vi "Fit.vi"(8 "error in (no error)":errorcluster caption="entrée d'erreur (pas d'erreur)", 9 "y":string[][](array[string]), 10 "X":string[][](array[string]), 11 "FunctionTransformer.lvclass":refnum<class "FunctionTransformer.lvclass">) -> (0 "error in (no error)":errorcluster caption="entrée d'erreur (pas d'erreur)", 2 "String Data":string, 3 "FunctionTransformer.lvclass":refnum<class "FunctionTransformer.lvclass">)   [LabVIEW 2020, in "FunctionTransformer.lvclass"]
doc: "Fit transformer by checking X.\n\nIf validate is True, X will be checked.\n\nReturns : \n\n- String : OK"
uses:
  FunctionTransformer.lvclass
  FunctionTransformer.lvclass/FunctionTransformer.ctl
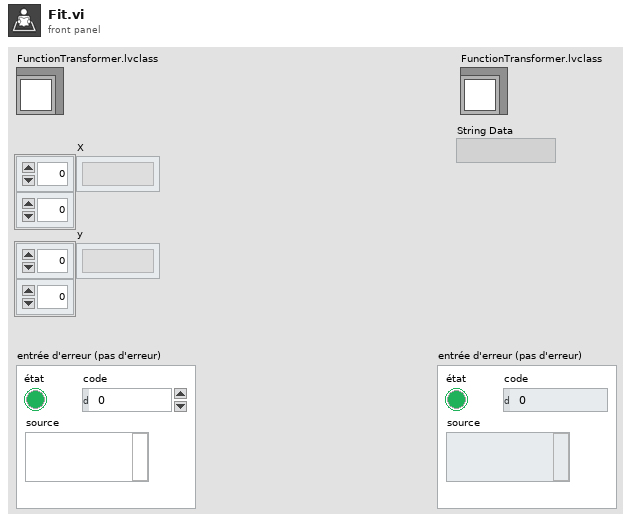
[diagram p1: front panel]
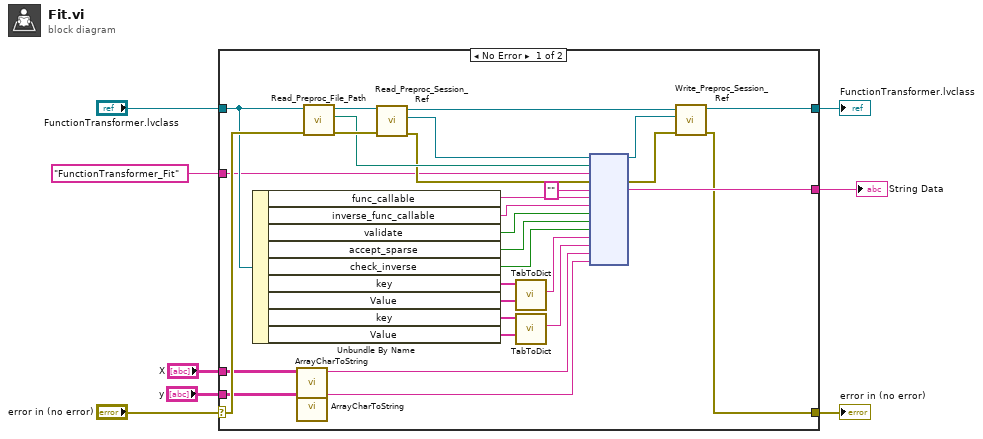
[diagram p0: block diagram]
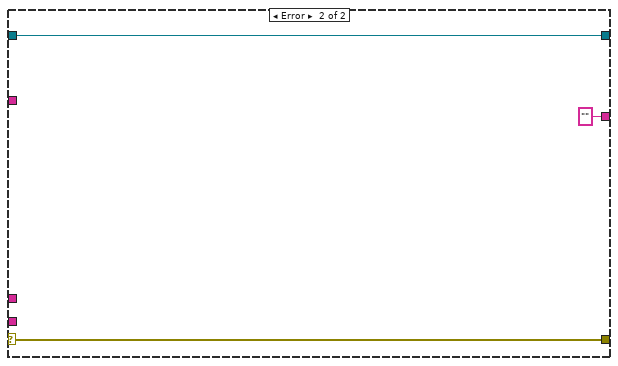
[diagram p2: hidden frame]
diagram:
  n1 = case shown="No Error" "error in (no error)" {
    selector: "error in (no error)" -> [w29 w41]
    tunnel: [w19 w41] -> w7
    tunnel: [w21 w40] -> w5
    tunnel: "FunctionTransformer.lvclass" -> [w28 w40]
    tunnel: "FunctionTransformer_Fit" ("Fonction") -> [w22 _]
    tunnel: [w20 ""] -> w3
    tunnel: "X" -> [w12 _]
    tunnel: "y" -> [w11 _]
    frame No Error {
      n2 = Unbundle By Name(w28) -> ("func_callable"=w27:string, "inverse_func_callable"=w26:string, "validate"=w25:bool, "accept_sparse"=w24:bool, "check_inverse"=w23:bool, "key"=w18:string[], "Value"=w17:string[], "key"=w16:string[], "Value"=w15:string[])
      n3 = call "ArrayCharToString.vi"("TAB"=w12) -> ("Instruction"=w10:string)  [unwired: 10 in]
      n4 = call "ArrayCharToString.vi"("TAB"=w11) -> ("Instruction"=w9:string)  [unwired: 10 in]
      n5 = call-dynamic "Read_Preproc_File_Path.vi"("error in (no error)"=w29, "Python in"=w28) -> ("error out"=w37:errorcluster, "File_Path"=w34:path, "Python out"=w38:refnum<class "FunctionTransformer.lvclass">)  [unwired: 7 in]
      n6 = call-dynamic "Read_Preproc_Session_Ref.vi"("error in (no error)"=w37, "Python in"=w38) -> ("error out"=w33:errorcluster, "Session_ref"=w35:refnum<k35>, "Python out"=w36:refnum<class "FunctionTransformer.lvclass">)  [unwired: 7 in]
      n7 = call "TabToDict.vi"("String Value"=w17, "String key"=w18) -> ("Dict with string value"=w13:string)  [unwired: 8 in, 1 out]
      n8 = call "TabToDict.vi"("String Value"=w15, "String key"=w16) -> ("Dict with string value"=w14:string)  [unwired: 8 in, 1 out]
      n9 = node(w35, w34, w22, w33, "", w27, w26, w25, w24, w23, w13, w14, w10, w9) -> (w31:refnum<k35>, w32:errorcluster, w20:string)  [unwired: 9 in, 2 out]
      n10 = call-dynamic "Write_Preproc_Session_Ref.vi"("error in (no error)"=w32, "Session_ref"=w31, "Python in"=w36) -> ("error out"=w19:errorcluster, "Python out"=w21:refnum<class "FunctionTransformer.lvclass">)  [unwired: 7 in]
    }
    frame Error {
    }
  }
  "error in (no error)" <- w7
  "FunctionTransformer.lvclass" <- w5
  "String Data" <- w3
